vi "scrap.vi"() -> (0 "Init Data Out":fxp<+/-,32,16>[][](array[numeric]))   [LabVIEW 2020]
panel:
  # "For Initialization VI requirements and help, please read directions located on Block Diagram."
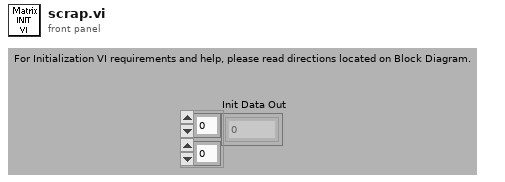
[diagram p1: front panel]
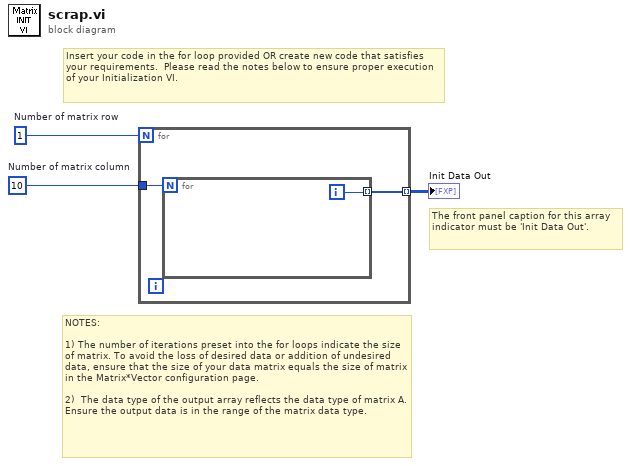
[diagram p0: block diagram]
diagram:
  w1 = 10  # Number of matrix column
  w3 = 1  # Number of matrix row
  # "The front panel caption for this array indicator must be 'Init Data Out'."
  # "NOTES:\n\n1) The number of iterations preset into the for loops indicate the size of matrix. To avoid the loss of desired data or addition of undesired data, ensure that the size of your data matrix equals the size of matrix in the Matrix*Vector configuration page.\n\n2)  The data type of the output array reflects the data type of matrix A.  Ensure the output data is in the range of the matrix data type."
  # "Insert your code in the for loop provided OR create new code that satisfies your requirements.  Please read the notes below to ensure proper execution of your Initialization VI."
  n1 = for {
    N: w3 -> [_]
    tunnel: [w5] -> w2 mode=indexing
    tunnel: w1 -> [w4]
    n2 = for {
      N: w4 -> [_]
      tunnel: [w6] -> w5 mode=indexing
      i -> [w6]
    }
  }
  "Init Data Out" <- w2
